vi "SettingsUpdate.vi"(8 "error in (no error)":errorcluster, 10 "Command":string, 11 "Control in":refnum<class "Control-Server.lvclass">) -> (0 "error out":errorcluster, 3 "Control out":refnum<class "Control-Server.lvclass">)   [LabVIEW 2020, in "Control-Server.lvclass"]
uses:
  Control-Server.lvclass
  Config/config_names_def.ctl
  Control-Server.lvclass/Control-Server.ctl
  GeneralFunctionality/GeneralFunctionality.lvclass/GeneralFunctionality.ctl
  Delay Line/DelayLine.lvclass
  C:/Dev/TRANCON/Classes/GeneralFunctionality/GeneralFunctionality.lvclass
  Detector/Detector.lvclass
  DAQmxTasks/DAQmxTaskContainer_General/DAQmxTaksContainer_General.lvclass
  Oscilloscope/Oscilloscope.lvclass
  Config/Config.lvclass
  GeneralFunctionality/GeneralFunctionality.lvclass
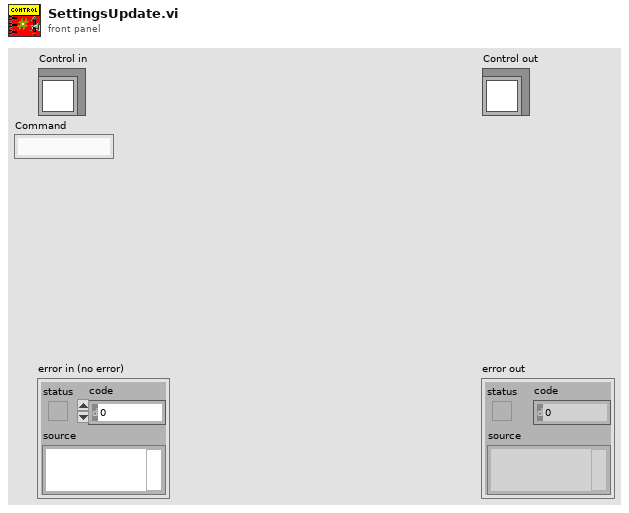
[diagram p1: front panel]
types:
  T1 = typedef "Config.lvclass/config_names_def.ctl" = string
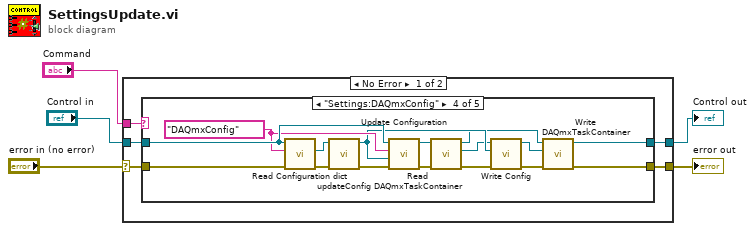
[diagram p0: block diagram]
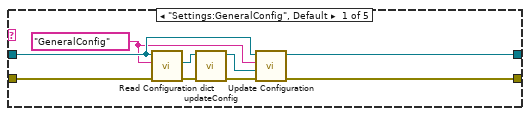
[diagram p2: hidden frame]
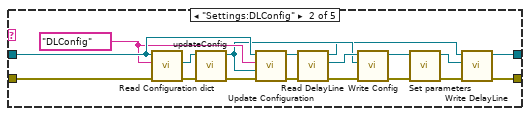
[diagram p3: hidden frame]
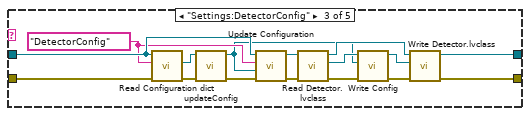
[diagram p4: hidden frame]
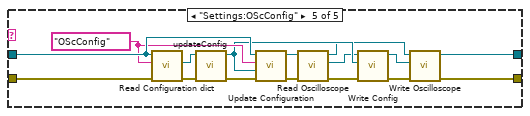
[diagram p5: hidden frame]
diagram:
  n1 = case shown="No Error" "error in (no error)" {
    selector: "error in (no error)" -> [w7 w87]
    tunnel: [w8 w87] -> w1
    tunnel: [w9 w86] -> w2
    tunnel: "Control in" -> [w10 w86]
    tunnel: "Command" -> [w6 _]
    frame No Error {
      n2 = case shown="\"Settings:DAQmxConfig\"" w6 {
        tunnel: w10 -> [w17 w36 w52 w68 w84]
        tunnel: w7 -> [w13 w33 w49 w65 w81]
        tunnel: [w14 w26 w39 w56 w72] -> w8
        tunnel: [w16 w27 w40 w57 w73] -> w9
        frame "Settings:GeneralConfig", Default {
          w11 = T1 "GeneralConfig" ("Config Name")
          n3 = call "Read Configuration dict.vi"("error in (no error)"=w13, "Config Name"=w11, "Control in"=w17) -> ("error out"=w12:errorcluster, "Config"=w19:refnum<class "Config.lvclass">)  [unwired: 6 in, 1 out]
          n4 = call "updateConfig.vi"("error in"=w12, "Config in"=w19) -> ("error out"=w15:errorcluster, "Config out"=w18:refnum<class "Config.lvclass">)  [unwired: 8 in]
          n5 = call "Update Configuration.vi"("error in (no error)"=w15, "Config.lvclass"=w18, "Config name"=w11, "Control in"=w17) -> ("error out"=w14:errorcluster, "Control out"=w16:refnum<class "Control-Server.lvclass">)  [unwired: 6 in]
        }
        frame "Settings:DLConfig" {
          w34 = T1 "DLConfig" ("Config Name")
          n6 = call "Read Configuration dict.vi"("error in (no error)"=w33, "Config Name"=w34, "Control in"=w36) -> ("error out"=w32:errorcluster, "Config"=w37:refnum<class "Config.lvclass">)  [unwired: 6 in, 1 out]
          n7 = call "updateConfig.vi"("error in"=w32, "Config in"=w37) -> ("error out"=w35:errorcluster, "Config out"=w29:refnum<class "Config.lvclass">)  [unwired: 8 in]
          n8 = call "Update Configuration.vi"("error in (no error)"=w35, "Config.lvclass"=w29, "Config name"=w34, "Control in"=w36) -> ("error out"=w24:errorcluster, "Control out"=w31:refnum<class "Control-Server.lvclass">)  [unwired: 6 in]
          n9 = call "Read DelayLine.vi"("error in (no error)"=w24, "Control in"=w31) -> ("error out"=w25:errorcluster, "DelayLine.lvclass"=w30:refnum<class "DelayLine.lvclass">, "Control out"=w28:refnum<class "Control-Server.lvclass">)  [unwired: 7 in]
          n10 = call "Write Config.vi"("error in (no error)"=w25, "Config.lvclass"=w29, "GeneralFunctionality en entrée"=w30) -> ("error out"=w23:errorcluster, "GeneralFunctionality en sortie"=w20:refnum<class "DelayLine.lvclass">)  [unwired: 7 in]
          n11 = call-dynamic "Set parameters.vi"("error in (no error)"=w23, "DelayLine en entrée"=w20) -> ("error out"=w22:errorcluster, "DelayLine en sortie"=w21:refnum<class "DelayLine.lvclass">)  [unwired: 8 in]
          n12 = call "Write DelayLine.vi"("error in (no error)"=w22, "DelayLine.lvclass"=w21, "Control in"=w28) -> ("error out"=w26:errorcluster, "Control out"=w27:refnum<class "Control-Server.lvclass">)  [unwired: 7 in]
        }
        frame "Settings:DetectorConfig" {
          w50 = T1 "DetectorConfig" ("Config Name")
          n13 = call "Read Configuration dict.vi"("error in (no error)"=w49, "Config Name"=w50, "Control in"=w52) -> ("error out"=w48:errorcluster, "Config"=w53:refnum<class "Config.lvclass">)  [unwired: 6 in, 1 out]
          n14 = call "updateConfig.vi"("error in"=w48, "Config in"=w53) -> ("error out"=w51:errorcluster, "Config out"=w44:refnum<class "Config.lvclass">)  [unwired: 8 in]
          n15 = call "Update Configuration.vi"("error in (no error)"=w51, "Config.lvclass"=w44, "Config name"=w50, "Control in"=w52) -> ("error out"=w38:errorcluster, "Control out"=w47:refnum<class "Control-Server.lvclass">)  [unwired: 6 in]
          n16 = call "Read Detector.lvclass.vi"("error in (no error)"=w38, "Control in"=w47) -> ("error out"=w43:errorcluster, "Detector.lvclass"=w45:refnum<class "Detector.lvclass">, "Control out"=w46:refnum<class "Control-Server.lvclass">)  [unwired: 7 in]
          n17 = call "Write Config.vi"("error in (no error)"=w43, "Config.lvclass"=w44, "GeneralFunctionality en entrée"=w45) -> ("error out"=w42:errorcluster, "GeneralFunctionality en sortie"=w41:refnum<class "Detector.lvclass">)  [unwired: 7 in]
          n18 = call "Write Detector.lvclass.vi"("error in (no error)"=w42, "Detector.lvclass"=w41, "Control in"=w46) -> ("error out"=w39:errorcluster, "Control out"=w40:refnum<class "Control-Server.lvclass">)  [unwired: 7 in]
        }
        frame "Settings:DAQmxConfig" {
          w66 = T1 "DAQmxConfig" ("Config Name")
          n19 = call "Read Configuration dict.vi"("error in (no error)"=w65, "Config Name"=w66, "Control in"=w68) -> ("error out"=w64:errorcluster, "Config"=w69:refnum<class "Config.lvclass">)  [unwired: 6 in, 1 out]
          n20 = call "updateConfig.vi"("error in"=w64, "Config in"=w69) -> ("error out"=w67:errorcluster, "Config out"=w63:refnum<class "Config.lvclass">)  [unwired: 8 in]
          n21 = call "Update Configuration.vi"("error in (no error)"=w67, "Config.lvclass"=w63, "Config name"=w66, "Control in"=w68) -> ("error out"=w61:errorcluster, "Control out"=w62:refnum<class "Control-Server.lvclass">)  [unwired: 6 in]
          n22 = call-dynamic "Read DAQmxTaskContainer.vi"("error in (no error)"=w61, "Control in"=w62) -> ("error out"=w59:errorcluster, "DAQmxTaksContainer_General.lvclass"=w60:refnum<class "DAQmxTaksContainer_General.lvclass">, "Control out"=w58:refnum<class "Control-Server.lvclass">)  [unwired: 7 in]
          n23 = call "Write Config.vi"("error in (no error)"=w59, "Config.lvclass"=w63, "GeneralFunctionality en entrée"=w60) -> ("error out"=w55:errorcluster, "GeneralFunctionality en sortie"=w54:refnum<class "DAQmxTaksContainer_General.lvclass">)  [unwired: 7 in]
          n24 = call-dynamic "Write DAQmxTaskContainer.vi"("error in (no error)"=w55, "DAQmxTaksContainer_General.lvclass"=w54, "Control in"=w58) -> ("error out"=w56:errorcluster, "Control out"=w57:refnum<class "Control-Server.lvclass">)  [unwired: 7 in]
        }
        frame "Settings:OScConfig" {
          w82 = T1 "OScConfig" ("Config Name")
          n25 = call "Read Configuration dict.vi"("error in (no error)"=w81, "Config Name"=w82, "Control in"=w84) -> ("error out"=w80:errorcluster, "Config"=w85:refnum<class "Config.lvclass">)  [unwired: 6 in, 1 out]
          n26 = call "updateConfig.vi"("error in"=w80, "Config in"=w85) -> ("error out"=w83:errorcluster, "Config out"=w79:refnum<class "Config.lvclass">)  [unwired: 8 in]
          n27 = call "Update Configuration.vi"("error in (no error)"=w83, "Config.lvclass"=w79, "Config name"=w82, "Control in"=w84) -> ("error out"=w77:errorcluster, "Control out"=w78:refnum<class "Control-Server.lvclass">)  [unwired: 6 in]
          n28 = call "Read Oscilloscope.vi"("error in (no error)"=w77, "Control-Server en entrée"=w78) -> ("error out"=w75:errorcluster, "Oscilloscope.lvclass"=w76:refnum<class "Oscilloscope.lvclass">, "Control-Server en sortie"=w74:refnum<class "Control-Server.lvclass">)  [unwired: 7 in]
          n29 = call "Write Config.vi"("error in (no error)"=w75, "Config.lvclass"=w79, "GeneralFunctionality en entrée"=w76) -> ("error out"=w71:errorcluster, "GeneralFunctionality en sortie"=w70:refnum<class "Oscilloscope.lvclass">)  [unwired: 7 in]
          n30 = call "Write Oscilloscope.vi"("error in (no error)"=w71, "Oscilloscope.lvclass"=w70, "Control-Server en entrée"=w74) -> ("error out"=w72:errorcluster, "Control-Server en sortie"=w73:refnum<class "Control-Server.lvclass">)  [unwired: 7 in]
        }
      }
    }
    frame Error {
    }
  }
  "error out" <- w1
  "Control out" <- w2
